vi "Random Task Name.vi"(8 "error in":errorcluster) -> (0 "error out":errorcluster, 2 "resulting string":string)   [LabVIEW 2018, in "Main.lvlib"]
uses:
  ADM/Main.lvlib
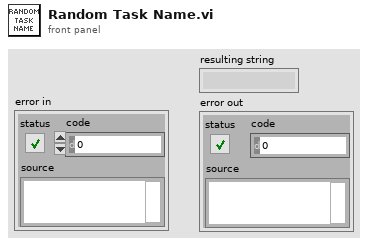
[diagram p1: front panel]
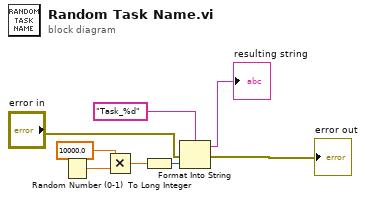
[diagram p0: block diagram]
diagram:
  n1 = Random Number (0-1)() -> (number: 0 to 1=w8:dbl)
  n2 = Multiply(x=10000.0, y=w8) -> (x*y=w6:dbl)
  n3 = To Long Integer(number=w6) -> (32bit integer=w5:i32)
  n4 = Format Into String(format string="Task_%d", error in="error in", w5) -> (resulting string=→"resulting string":string, error out=→"error out":errorcluster)  [unwired: 1 in]
